vi "Thingworx_Write_Bool.vi"(9 "Boolean":bool, 11 "Thingworx":string(xcontrol)) -> ()   [LabVIEW 2022 SP3]
uses:
  TW_XControl.xctl
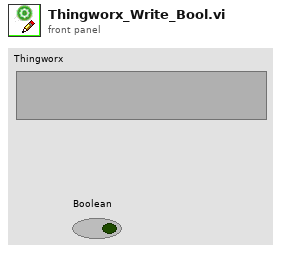
[diagram p1: front panel]
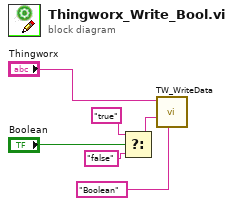
[diagram p0: block diagram]
diagram:
  n1 = Select(t="true", s="Boolean", f="false") -> (s? t:f=w2:string)
  n2 = call "TW_WriteData.vi"("Type"="Boolean", "value"=w2, "Property"="Thingworx") -> ()  [unwired: 9 in]
